vi "Translator.File.GetDefaultStrings.vi"   [LabVIEW 2010]
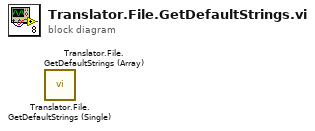
[diagram p0: block diagram]
diagram:
  n1 = call "Translator.File.GetDefaultStrings (Single).vi"() -> ()  [unwired: 10 in, 2 out]
  n2 = call "Translator.File.GetDefaultStrings (Array).vi"() -> ()  [unwired: 10 in, 2 out]
